vi "Ideal Gas Law calculator.vi"() -> ()   [LabVIEW 2024]
panel:
  in  "CASE SELECTION":T1(radio)
  out "Temperature Output\n(in Kelvin)":dbl format="%#_5g"
  out "Volume Output \n(in Cubic meters)":dbl format="%#_5g"
  out "Pressure Output \n(in Pascals)":dbl format="%#_5g"
  out "Thermometer":dbl(slide) scale=0.0..500.0 scale format="%#_5g"
  out "Volumeter":dbl(slide) scale=0.0..1000.0
  out "Pressure Gauge":dbl(knob) scale=0.0..1000.0
  in  "Input Controls":T2 {"No of Moles Input\n(integer)" min=0.0 format="%#_5g"; "Temperature Input\n(in Kelvin)" min=0.0 max=1000.0 format="%#_5g"; "Volume Input \n(in Cubic meters)" min=0.0 max=1000.0 format="%#_5g"; "Pressure Input \n(in Pascals)" min=0.0 max=1000.0 step=1.0 format="%#_5g"}
  # "IDEAL GAS LAW - CALCULATOR APP"
  # "PV = n*R*T"
  # "Ideal Gas Constant\nR = 8.314 J/(mol*K)"
  # "OUTPUT"
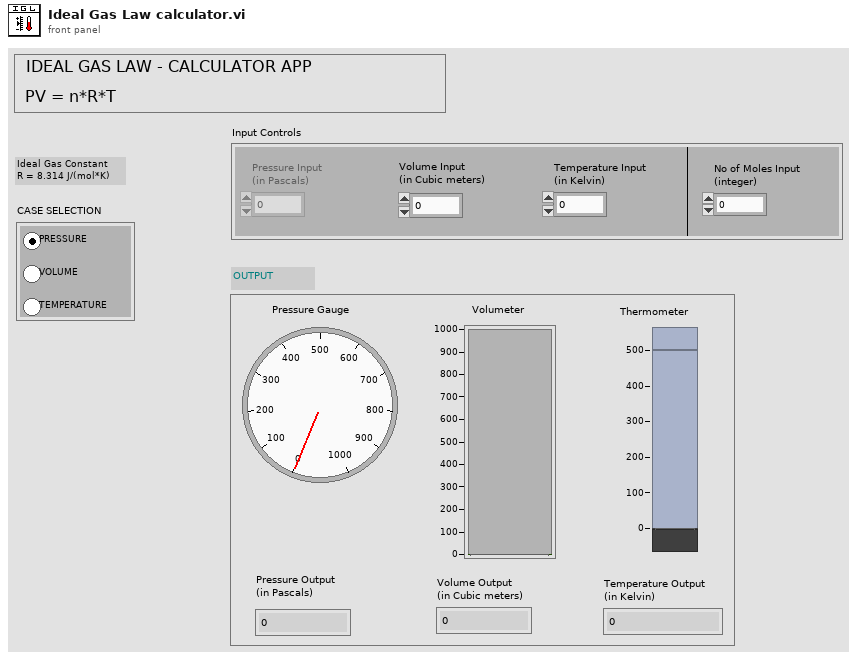
[diagram p1: front panel]
types:
  T1 = enum32{"1: Pressure", "2: Volume", "3: Temperature"}
  T2 = cluster{"Pressure Input \n(in Pascals)":dbl, "Volume Input \n(in Cubic meters)":dbl, "Temperature Input\n(in Kelvin)":dbl, "No of Moles Input\n(integer)":dbl}
  T3 = enum8{"Enabled", "Disabled", "Disabled and Grayed Out"}
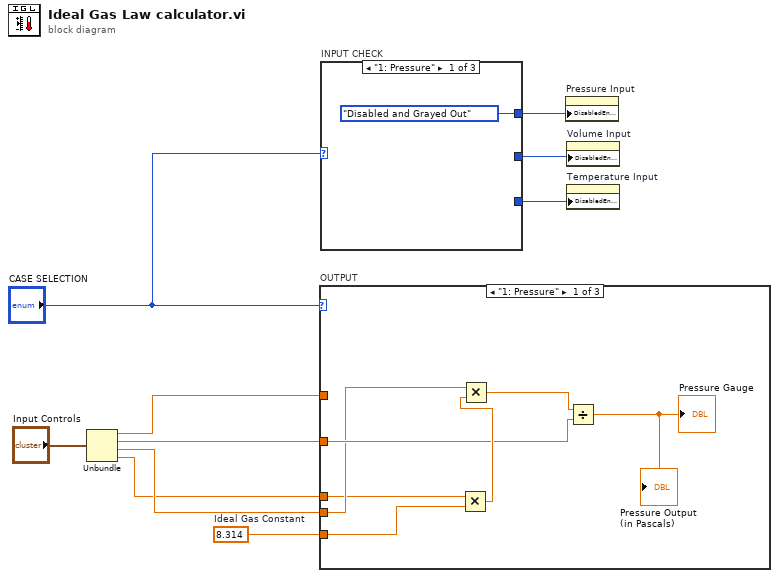
[diagram p0: block diagram]
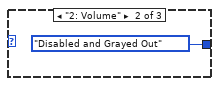
[diagram p2: hidden frame]
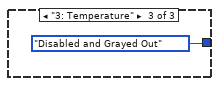
[diagram p3: hidden frame]
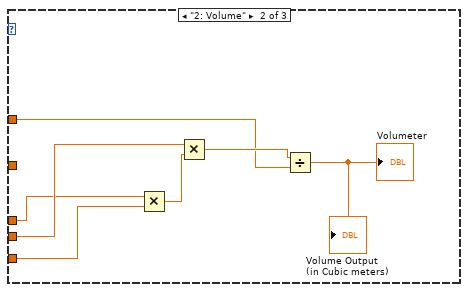
[diagram p4: hidden frame]
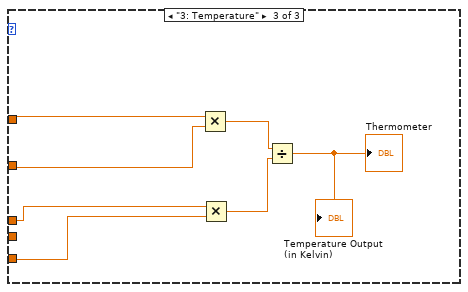
[diagram p5: hidden frame]
diagram:
  w6 = 8.314  # Ideal Gas Constant
  n1 = Unbundle("Input Controls") -> ("Pressure Input \n(in Pascals)"=w9:dbl, "Volume Input \n(in Cubic meters)"=w8:dbl, "Temperature Input\n(in Kelvin)"=w7:dbl, "No of Moles Input\n(integer)"=w5:dbl)
  n2 = case "OUTPUT" shown="\"1: Pressure\"" "CASE SELECTION" {
    tunnel: w9 -> [_ w20 w28]
    tunnel: w8 -> [w15 _ w29]
    tunnel: w7 -> [w13 w22 _]
    tunnel: w5 -> [w12 w19 w26]
    tunnel: w6 -> [w11 w18 w25]
    frame "1: Pressure" {
      n3 = Multiply(x=w12, y=w11) -> (x*y=w17:dbl)
      n4 = Multiply(x=w13, y=w17) -> (x*y=w16:dbl)
      n5 = Divide(x=w16, y=w15) -> (x/y=→"Pressure Gauge" →"Pressure Output \n(in Pascals)":dbl)
    }
    frame "2: Volume" {
      n6 = Multiply(x=w19, y=w18) -> (x*y=w24:dbl)
      n7 = Multiply(x=w22, y=w24) -> (x*y=w21:dbl)
      n8 = Divide(x=w21, y=w20) -> (x/y=→"Volumeter" →"Volume Output \n(in Cubic meters)":dbl)
    }
    frame "3: Temperature" {
      n9 = Multiply(x=w28, y=w29) -> (x*y=w31:dbl)
      n10 = Multiply(x=w26, y=w25) -> (x*y=w30:dbl)
      n11 = Divide(x=w31, y=w30) -> (x/y=→"Thermometer" →"Temperature Output\n(in Kelvin)":dbl)
    }
  }
  n12 = case "INPUT CHECK" shown="\"1: Pressure\"" "CASE SELECTION" {
    tunnel: [T3."Disabled and Grayed Out" ("Disabled") _ _] -> w3
    tunnel: [_ T3."Disabled and Grayed Out" ("Disabled") _] -> w2
    tunnel: [_ _ T3."Disabled and Grayed Out" ("Disabled")] -> w1
    frame "1: Pressure" {
    }
    frame "2: Volume" {
    }
    frame "3: Temperature" {
    }
  }
  n13 = property on="Pressure Input" class="DigNum (strict)"("DisabledEnum"=w3) -> ()  [unwired: 2 in, 2 out]
  n14 = property on="Volume Input" class="DigNum (strict)"("DisabledEnum"=w2) -> ()  [unwired: 2 in, 2 out]
  n15 = property on="Temperature Input" class="DigNum (strict)"("DisabledEnum"=w1) -> ()  [unwired: 2 in, 2 out]
